vi "Construct Stream To Disk Transport.vi"(10 "Channel Name":string, 11 "File Path":path) -> (0 "error out":errorcluster, 3 "StreamToDiskTransport":refnum<class "StreamToDiskTransport.lvclass">)   [LabVIEW 2020, in "StreamToDiskTransport.lvclass"]
doc: "<License>\nCopyright © 2017 Composed Systems, LLC | All rights reserved\nwww.composed.io\n\nAuthor: Ethan Stern <ethan.stern@composed.io>\n\nThis software is provided \"AS IS\" WITHOUT WARRANTIES, either express or implied, AND IS FOR EDUCATIONAL PURPOSES ONLY.\n</License>"
uses:
  <vilib>/gpm_packages/@cs/transport/Source/Concrete/StreamToDiskTransport/StreamToDiskTransport.lvclass
  <vilib>/gpm_packages/@cs/transport/Source/Concrete/StreamToDiskTransport/StreamToDiskTransport.lvclass/StreamToDiskTransport.ctl
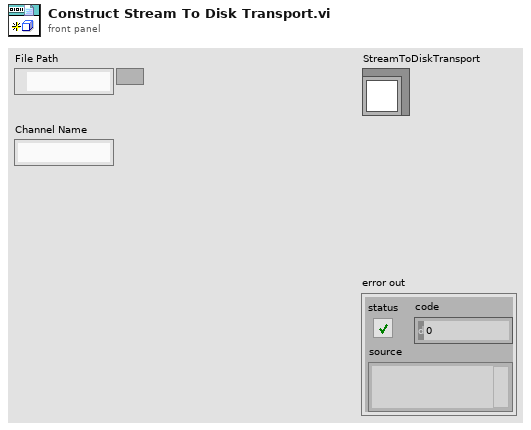
[diagram p1: front panel]
types:
  T1 = enum16{"open", "open or create", "create or replace", "create", "open (read-only)"}
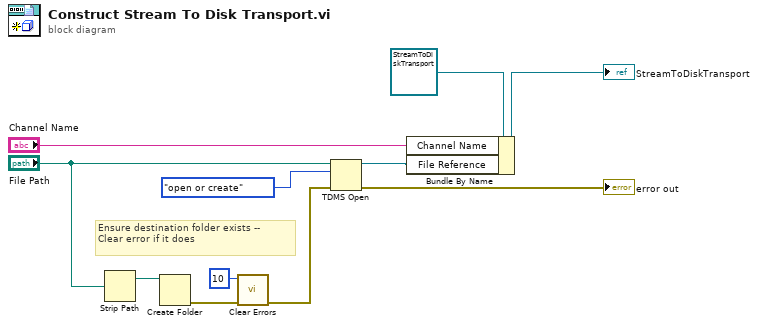
[diagram p0: block diagram]
diagram:
  # "Ensure destination folder exists --\nClear error if it does"
  n1 = Strip Path(path="File Path") -> (stripped path=w6:path)  [unwired: 1 out]
  n2 = Create Folder(path (use dialog)=w6) -> (error out=w5:errorcluster)  [unwired: 2 in, 2 out]
  n3 = call <vilib>:"Clear Errors.vi"("error in (no error)"=w5, "specific error code to clear (0: all)"=10) -> ("error out"=w3:errorcluster)  [unwired: 4 in, 1 out]
  n4 = TDMS Open(8:w3, 10:T1."open or create" ("operation (0:open)"), 11:"File Path") -> (0:→"error out":errorcluster, 3:w10:refnum<k34>)  [unwired: 4 in]
  n5 = Bundle By Name(cluster=refnum<class "StreamToDiskTransport.lvclass"> refnum ("StreamToDiskTransport"), "Channel Name"="Channel Name", "File Reference"=w10) -> (→"StreamToDiskTransport":refnum<class "StreamToDiskTransport.lvclass">)
